vi "GenerateJsonFileName.vi"(8 "Error In":errorcluster, 11 "Asset":refnum<class "Asset.lvclass">) -> (0 "Error Out":errorcluster, 3 "File Name":string)   [LabVIEW 2019, in "Asset.lvclass"]
uses:
  Asset/Asset.lvclass
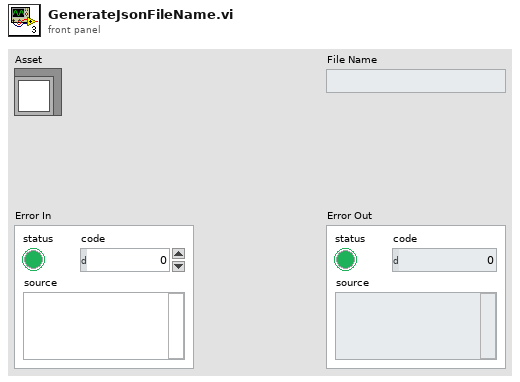
[diagram p1: front panel]
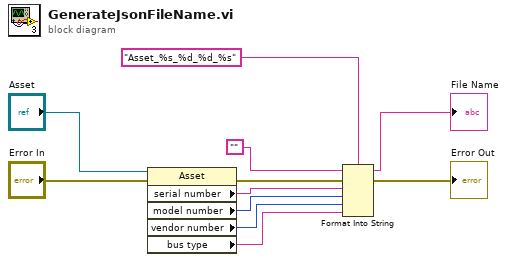
[diagram p0: block diagram]
diagram:
  n1 = property class="Asset"(reference="Asset", error in="Error In") -> (error out=w6:errorcluster, "serial number"=w5:string, "model number"=w4:u32, "vendor number"=w3:u32, "bus type"=w2:string)  [unwired: 1 out]
  n2 = Format Into String(format string="Asset_%s_%d_%d_%s" ("time format string (%c)"), initial string="", error in=w6, w5, w4, w3, w2) -> (resulting string=→"File Name":string, error out=→"Error Out":errorcluster)
